vi "profile_time.vi"(7 "Motor Adress":T1(ring)=enum."3", 8 "error in (no error)":errorcluster, 11 "VISA ressource in":refnum<visa-resource-name>="COM7") -> (0 "error out":errorcluster={"status"=FALSE, "code"=1073676294, "source"="VISA Read in write_read.vi"}, 1 "profile time (in ms)":u32, 2 "direction":i32, 3 "VISA ressource out":refnum<visa-resource-name>, 5 "steps":u32)   [LabVIEW 2013]
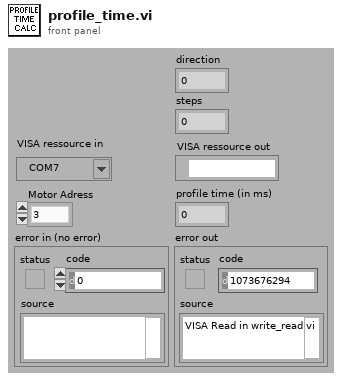
[diagram p1: front panel]
types:
  T1 = enum16{"All", "1", "2", "3", "4", "5", "6", "7", "8"}
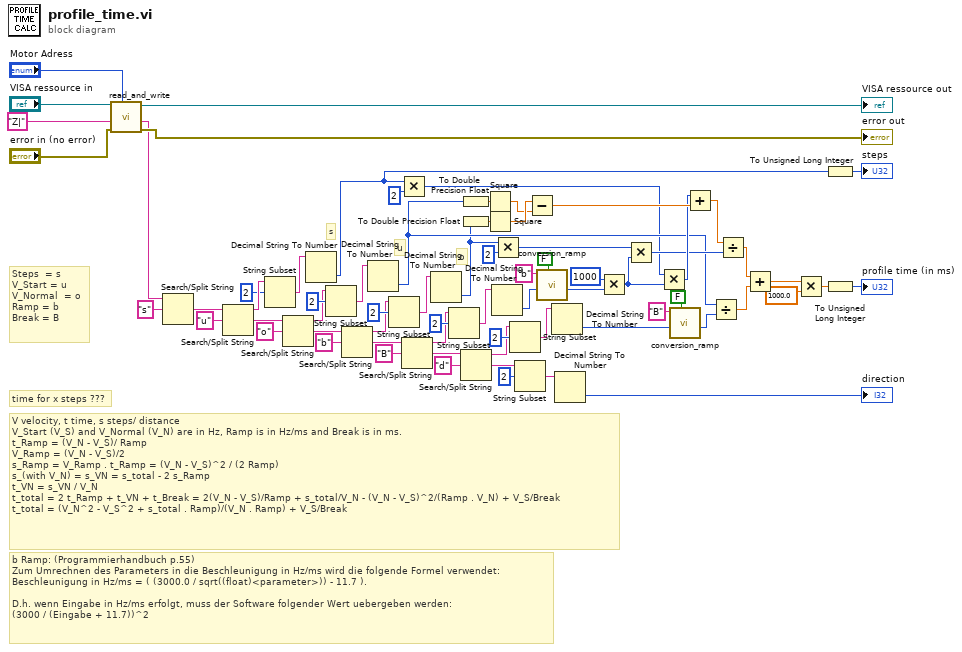
[diagram p0: block diagram]
diagram:
  # "o"
  # "u"
  # "s"
  # "b Ramp: (Programmierhandbuch p.55)\nZum Umrechnen des Parameters in die Beschleunigung in Hz/ms wird die folgende Formel verwendet:\nBeschleunigung in Hz/ms = ( (3000.0 / sqrt((float)<parameter>)) - 11.7 ).\n\nD.h. wenn Eingabe in Hz/ms erfolgt, muss der Software folgender Wert uebergeben werden:\n(3000 / (Eingabe + 11.7))^2"
  # "V velocity, t time, s steps/ distance\nV_Start (V_S) and V_Normal (V_N) are in Hz, Ramp is in Hz/ms and Break is in ms.\nt_Ramp = (V_N - V_S)/ Ramp\nV_Ramp = (V_N - V_S)/2\ns_Ramp = V_Ramp . t_Ramp = (V_N - V_S)^2 / (2 Ramp)\ns_(with V_N) = s_VN = s_total - 2 s_Ramp\nt_VN = s_VN / V_N\nt_total = 2 t_Ramp + t_VN + t_Break = 2(V_N - V_S)/Ramp + s_total/V_N - (V_N - V_S)^2/(Ramp . V_N) + V_S/Break\nt_total = (V_N^2 - V_S^2 + s_total . Ramp)/(V_N . Ramp) + V_S/Break"
  # "time for x steps ???"
  # "Steps  = s\nV_Start = u \nV_Normal  = o\nRamp = b\nBreak = B"
  n1 = call "read_and_write.vi"("Motor Adress"="Motor Adress", "error in (no error)"="error in (no error)", "Command"="Z|", "VISA ressource in"="VISA ressource in") -> ("error out"=→"error out":errorcluster, "Answer"=w66:string, "VISA ressource out"=→"VISA ressource out":refnum<visa-resource-name>)  [unwired: 4 in, 1 out]
  n2 = Search/Split String(string=w66, search string/char (-)="s") -> (match + rest of string=w60:string)  [unwired: 1 in, 2 out]
  n3 = Search/Split String(string=w60, search string/char (-)="u") -> (substring before match=w54:string, match + rest of string=w59:string)  [unwired: 1 in, 1 out]
  n4 = String Subset(string=w54, offset (0)=2) -> (substring=w42:string)  [unwired: 1 in]
  n5 = Search/Split String(string=w59, search string/char (-)="o") -> (substring before match=w46:string, match + rest of string=w58:string)  [unwired: 1 in, 1 out]
  n6 = Decimal String To Number(string=w42) -> (number=w10:i32)  [unwired: 2 in, 1 out]
  n7 = String Subset(string=w46, offset (0)=2) -> (substring=w41:string)  [unwired: 1 in]
  n8 = Search/Split String(string=w58, search string/char (-)="b") -> (substring before match=w45:string, match + rest of string=w57:string)  [unwired: 1 in, 1 out]
  n9 = Decimal String To Number(string=w41) -> (number=w15:i32)  [unwired: 2 in, 1 out]
  n10 = String Subset(string=w45, offset (0)=2) -> (substring=w40:string)  [unwired: 1 in]
  n11 = Multiply(x=w10, y=2) -> (x*y=w9:i32)
  n12 = Search/Split String(string=w57, search string/char (-)="B") -> (substring before match=w44:string, match + rest of string=w55:string)  [unwired: 1 in, 1 out]
  n13 = Decimal String To Number(string=w40) -> (number=w8:i32)  [unwired: 2 in, 1 out]
  n14 = String Subset(string=w44, offset (0)=2) -> (substring=w39:string)  [unwired: 1 in]
  n15 = To Double Precision Float(number=w15) -> (double precision float=w2:dbl)
  n16 = To Double Precision Float(number=w8) -> (double precision float=w1:dbl)
  n17 = Search/Split String(string=w55, search string/char (-)="d") -> (substring before match=w43:string, match + rest of string=w20:string)  [unwired: 1 in, 1 out]
  n18 = Square(x=w2) -> (x^2=w30:dbl)
  n19 = Square(x=w1) -> (x^2=w31:dbl)
  n20 = Decimal String To Number(string=w39) -> (number=w34:i32)  [unwired: 2 in, 1 out]
  n21 = Multiply(x=w8, y=2) -> (x*y=w6:i32)
  n22 = String Subset(string=w43, offset (0)=2) -> (substring=w38:string)  [unwired: 1 in]
  n23 = String Subset(string=w20, offset (0)=2) -> (substring=w19:string)  [unwired: 1 in]
  n24 = Subtract(x=w31, y=w30) -> (x-y=w29:dbl)
  n25 = call "conversion_ramp.vi"("From Hz/ms to Driver"=FALSE, "Value"=w34, "Command"="b") -> ("Value out"=w5:i32)  [unwired: 7 in, 1 out]
  n26 = Decimal String To Number(string=w38) -> (number=w22:i32)  [unwired: 2 in, 1 out]
  n27 = Decimal String To Number(string=w19) -> (number=→"direction":i32)  [unwired: 2 in, 1 out]
  n28 = Multiply(x=1000, y=w5) -> (x*y=w3:i32)
  n29 = Multiply(x=w6, y=w3) -> (x*y=w26:i32)
  n30 = Multiply(x=w9, y=w3) -> (x*y=w28:i32)
  n31 = call "conversion_ramp.vi"("From Hz/ms to Driver"=FALSE, "Value"=w22, "Command"="B") -> ("Value out"=w17:i32)  [unwired: 7 in, 1 out]
  n32 = Add(x=w28, y=w29) -> (x+y=w27:dbl)
  n33 = Divide(x=w15, y=w17) -> (x/y=w16:dbl)
  n34 = Divide(x=w27, y=w26) -> (x/y=w25:dbl)
  n35 = Add(x=w25, y=w16) -> (x+y=w14:dbl)
  n36 = Multiply(x=w14, y=1000.0) -> (x*y=w12:dbl)
  n37 = To Unsigned Long Integer(number=w10) -> (unsigned 32bit integer=→"steps":u32)
  n38 = To Unsigned Long Integer(number=w12) -> (unsigned 32bit integer=→"profile time (in ms)":u32)
